vi "Fuel Injector Analysis Selection.vi"(8 "error in (no error)":errorcluster, 11 "Node Ptr":T1 format="%.0x") -> (0 "error out":errorcluster)   [LabVIEW 2019, in "Fuel Injector Analysis Addon System Explorer.lvlib"]
uses:
  Fuel Injector Analysis Addon System Explorer.lvlib
  <vilib>/NI VeriStand/Custom Device API/Custom Device Item Ref.ctl
  Addon Shared/Types/Analysis.Channels.Select.ctl
  <vilib>/NI VeriStand/Custom Device API/Custom Device API.lvlib
  Addon Shared/Fuel Injector Analysis Addon Shared.lvlib
panel:
  in  "Analysis":i32(listbox)=7
  in  "Reset":bool
  in  "Apply":bool
  in  "SHDocVw.IWebBrowser":refnum<k7>(container)
  in  "Header":cluster{"Section Name":string}={"Section Name"="Custom Device Item Settings"}
  in  "Description":string
  out "Name":string
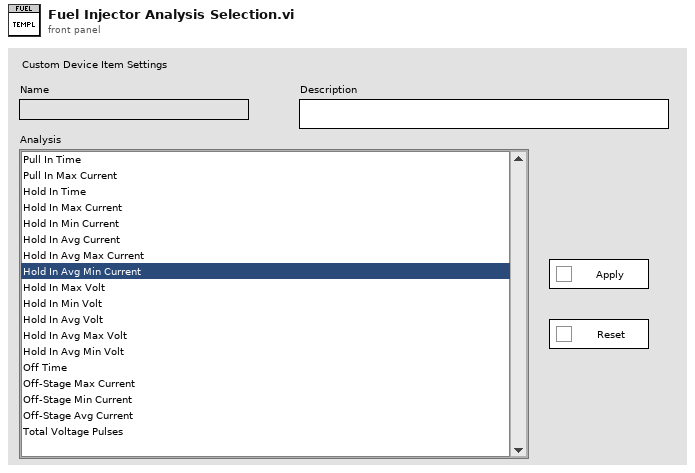
[diagram p1: front panel]
types:
  T1 = typedef "Custom Device API.lvlib/Custom Device Item Ref.ctl" = u64
  T2 = typedef "Custom Device API.lvlib/Custom Device Item Info.ctl" = cluster{"Name":string, "Is Channel":bool, "GUID":string, "Is Waveform":bool}
  T3 = typedef "Fuel Injector Analysis Addon Shared.lvlib/Analysis.Channels.Select.ctl" = cluster{"Pull In Time":bool, "Pull In Max Current":bool, "Pull In Max Voltage":bool, "Pull In Min Voltage":bool, "Pull In Avg Voltage":bool, "Hold Time":bool, "Hold Max Current":bool, "Hold Min Current":bool, "Hold Avg Current":bool, "Hold Max Voltage":bool, "Hold Min Voltage":bool, "Hold Avg Max Voltage":bool, "Hold Avg Min Voltage":bool, "Off Time":bool, "Off Max Current":bool, "Off Min Current":bool, "Off Avg Current":bool, "Off Max Voltage":bool, "Off Min Voltage":bool, "Off Avg Voltage":bool, "Total Voltage Pulses":bool, "Total Stage Time":bool}
  T4 = typedef "Custom Device API.lvlib/Custom Device Commands.ctl" = enum16{"Default", "Item renamed", "Shutdown", "Dynamic button pressed"}
  T5 = typedef "LVPoint32TypeDef.ctl" = cluster{"Horizontal":i32, "Vertical":i32}
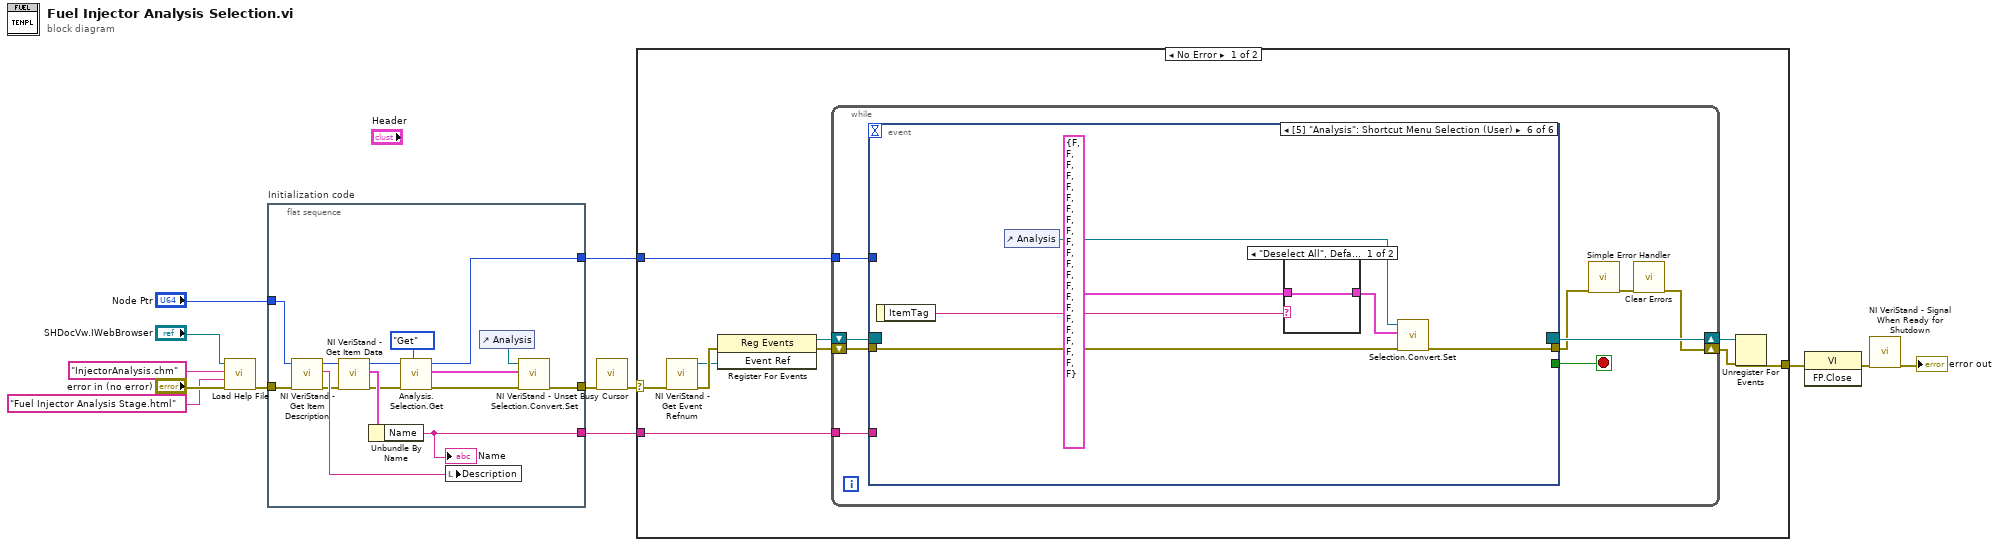
[diagram p0: block diagram]
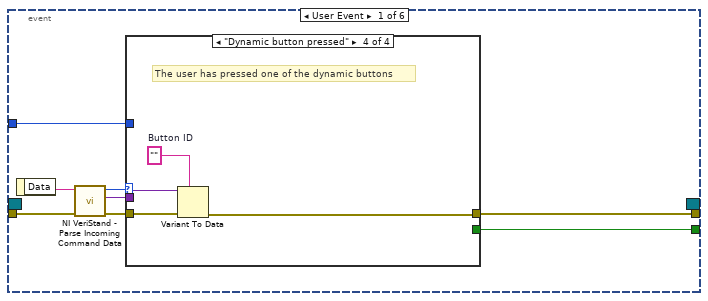
[diagram p2: hidden frame]
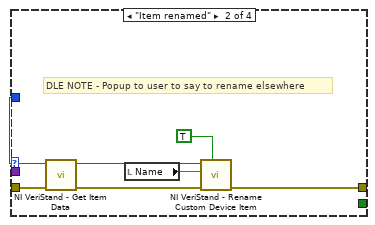
[diagram p4: hidden frame]
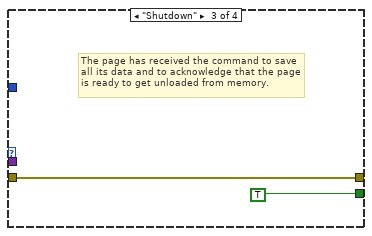
[diagram p5: hidden frame]
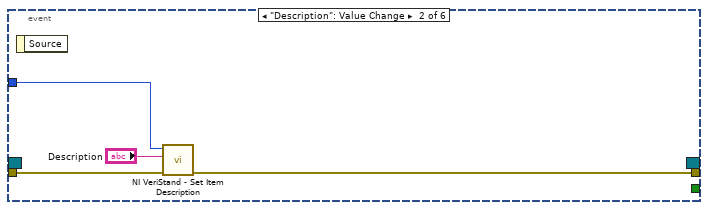
[diagram p6: hidden frame]
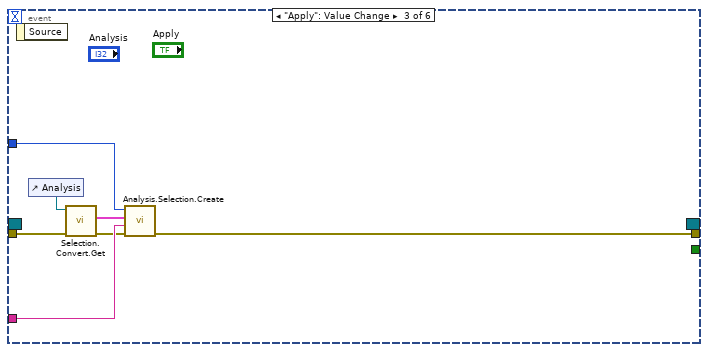
[diagram p7: hidden frame]
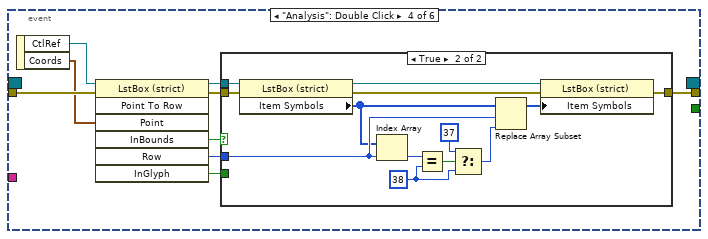
[diagram p8: hidden frame]
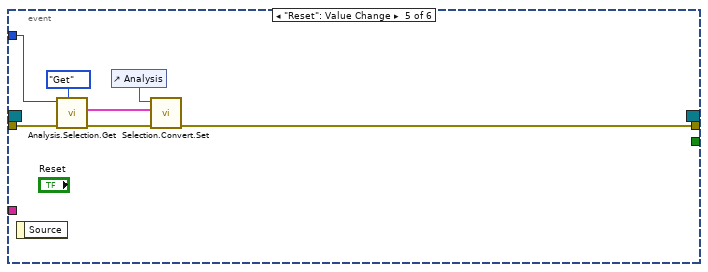
[diagram p10: hidden frame]
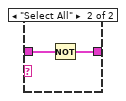
[diagram p11: hidden frame]
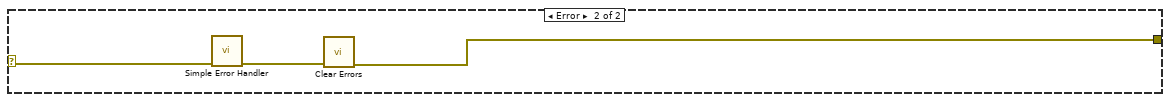
[diagram p12: hidden frame]
diagram:
  n1 = call "Load Help File.vi"("error in (no error)"="error in (no error)", "HTML File"="Fuel Injector Analysis Stage.html", "Main CHM File"="InjectorAnalysis.chm", "SHDocVw.IWebBrowser2"="SHDocVw.IWebBrowser") -> ("error out"=w6:errorcluster)  [unwired: 7 in]
  n2 = flat-sequence "Initialization code" {
    tunnel: w6 -> [w27]
    tunnel: [w15] -> w9
    tunnel: "Node Ptr" -> [w23]
    tunnel: [w20] -> w3
    tunnel: [w14] -> w2
    frame #0 {
      n3 = call <vilib>:"NI VeriStand - Get Item Description.vi"("error in (no error)"=w27, "Item Ref in"=w23) -> ("error out"=w25:errorcluster, "Description"=w26:string, "Item Ref out"=w28:T1)  [unwired: 7 out]
      n4 = call <vilib>:"NI VeriStand - Get Item Data.vi"("error in (no error)"=w25, "Item Ref in"=w28) -> ("error out"=w22:errorcluster, "Item Info"=w24:T2, "Item Ref out"=w21:T1)  [unwired: 7 out]
      n5 = Unbundle By Name(w24) -> ("Name"=w20:string)
      "Name" <- w20
      n6 = call "Analysis.Selection.Get.vi"("Action"=enum8{"Get", "Set"}."Get", "error in (no error)"=w22, "Item Ref in"=w21) -> ("error out"=w17:errorcluster, "Selections"=w18:T3, "Item Ref out"=w15:T1)  [unwired: 6 in]
      n7 = local write "Description"(w26) -> ()
      n8 = control-ref of="Analysis"() -> (w16:refnum<vi>)
      n9 = call "Selection.Convert.Set.vi"("error in (no error)"=w17, "Selections"=w18, "ListBox in"=w16) -> ("error out"=w14:errorcluster)  [unwired: 8 in]
    }
  }
  n10 = call <vilib>:"NI VeriStand - Unset Busy Cursor.vi"("error in (no error)"=w2) -> ("error out"=w10:errorcluster)  [unwired: 10 out]
  n11 = case shown="No Error" w10 {
    selector: w10 -> [w30 w122]
    tunnel: [w35 w120] -> w13
    tunnel: w9 -> [w31 _]
    tunnel: w3 -> [w29 _]
    frame No Error {
      n12 = call <vilib>:"NI VeriStand - Get Event Refnum.vi"("error in (no error)"=w30) -> ("error out"=w38:errorcluster, "Event Ref"=w34:refnum<user-event>)  [unwired: 9 out]
      n13 = register-events(error in=w38, w34) -> (reference out=w32:refnum<event-registration>, error out=w33:errorcluster)  [unwired: 1 in]
      n14 = while {
        tunnel: w31 -> [w43]
        shift-right: [w40] -> w36
        shift-left: w33 -> [w46]
        shift-right: [w47] -> w37
        shift-left: w32 -> [w45]
        tunnel: w29 -> [w39]
        stop <- w44 stop-if-true
        n15 = event shown="[5] \"Analysis\": Shortcut Menu Selection (User)" {
          selector: w45 -> [_ _ _ _ _ _]
          dyn-events: [_ _ _ _ _ _] -> w47
          timeout: _ -> [_ _ _ _ _ _]
          tunnel: w46 -> [w55 w72 w78 w83 w105 w114]
          tunnel: [w51 _ _ _ _ _] -> w44
          tunnel: [w50 w71 w74 w81 w107 w113] -> w42
          tunnel: w43 -> [w49 w73 w79 _ w104 _]
          tunnel: w39 -> [_ _ w80 _ _ _]
          event User Event {
            n16 = event-data() -> ("Data"=w54:string)  [unwired: 1 out]
            n17 = call <vilib>:"NI VeriStand - Parse Incoming Command Data.vi"("error in (no error)"=w55, "Incoming data"=w54) -> ("error out"=w53:errorcluster, "Outgoing data"=w48:variant, "Action"=w52:T4)  [unwired: 7 out]
            n18 = case shown="\"Dynamic button pressed\"" w52 {
              tunnel: w53 -> [w56 w63 w64 w69]
              tunnel: [_ _ TRUE _] -> w51
              tunnel: [w56 w60 w64 w66] -> w50
              tunnel: w49 -> [_ w62 _ _]
              tunnel: w48 -> [_ _ _ w68]
              frame "Default", Default {
              }
              frame "Item renamed" {
                # "DLE NOTE - Popup to user to say to rename elsewhere"
                n19 = call <vilib>:"NI VeriStand - Get Item Data.vi"("error in (no error)"=w63, "Item Ref in"=w62) -> ("error out"=w61:errorcluster, "Item Ref out"=w59:T1)  [unwired: 8 out]
                n20 = local read "Name"() -> (w58:string)
                n21 = call <vilib>:"NI VeriStand - Rename Custom Device Item.vi"("Force Rename (F)"=TRUE, "error in (no error)"=w61, "New Name"=w58, "Item Ref in"=w59) -> ("error out"=w60:errorcluster)  [unwired: 5 in, 2 out]
              }
              frame "Shutdown" {
                # "The page has received the command to save all its data and to acknowledge that the page is ready to get unloaded from memory."
              }
              frame "Dynamic button pressed" {
                w67 = ""  # Button ID
                # "The user has pressed one of the dynamic buttons"
                n22 = Variant To Data(error in=w69, type=w67, Variant=w68) -> (error out=w66:errorcluster)  [unwired: 1 out]
              }
            }
          }
          event "Description": Value Change {
            n23 = event-data() -> ()  [unwired: 2 out]
            n24 = call <vilib>:"NI VeriStand - Set Item Description.vi"("error in (no error)"=w72, "Description"="Description", "Item Ref in"=w73) -> ("error out"=w71:errorcluster)  [unwired: 8 out]
          }
          event "Apply": Value Change {
            n25 = event-data() -> ()  [unwired: 2 out]
            n26 = control-ref of="Analysis"() -> (w75:refnum<vi>)
            n27 = call "Selection.Convert.Get.vi"("error in (no error)"=w78, "ListBox in"=w75) -> ("error out"=w77:errorcluster, "Analysis Options"=w76:T3)  [unwired: 8 in]
            n28 = call "Analysis.Selection.Create.vi"("error in (no error)"=w77, "Name"=w80, "Analysis Options"=w76, "Item Ref in"=w79) -> ("error out"=w74:errorcluster)  [unwired: 7 in]
          }
          event "Analysis": Double Click {
            n29 = event-data() -> ("CtlRef"=w84:refnum<vi>, "Coords"=w82:T5)  [unwired: 1 out]
            n30 = invoke class="LstBox (strict)" method="Point To Row"(reference=w84, error in=w83, "Point"=w82) -> (reference out=w88:refnum<vi>, error out=w87:errorcluster, "InBounds"=w85:bool, "Row"=w86:i32, "InGlyph"=w89:bool)  [unwired: 4 in, 2 out]
            n31 = case shown="True" w85 {
              tunnel: w89 -> [_ _]
              tunnel: w88 -> [_ w103]
              tunnel: w87 -> [w90 w102]
              tunnel: w86 -> [_ w101]
              tunnel: [w90 w91] -> w81
              frame False {
              }
              frame True {
                w98 = 38
                n32 = property class="LstBox (strict)"(reference=w103, error in=w102) -> (reference out=w94:refnum<vi>, error out=w93:errorcluster, "Item Symbols"=w96:i32[])
                n33 = Index Array(array=w96, index=w101) -> (element=w100:i32)
                n34 = Equal?(x=w100, y=w98) -> (x = y?=w99:bool)
                n35 = Select(t=37, s=w99, f=w98) -> (s? t:f=w95:i32)
                n36 = Replace Array Subset(array=w96, new element=w95, index=w101) -> (w92:i32[])
                n37 = property class="LstBox (strict)"(reference=w94, error in=w93, "Item Symbols"=w92) -> (error out=w91:errorcluster)  [unwired: 1 out]
              }
            }
          }
          event "Reset": Value Change {
            n38 = event-data() -> ()  [unwired: 2 out]
            n39 = call "Analysis.Selection.Get.vi"("Action"=enum8{"Get", "Set"}."Get", "error in (no error)"=w105, "Item Ref in"=w104) -> ("error out"=w108:errorcluster, "Selections"=w106:T3)  [unwired: 6 in, 1 out]
            n40 = control-ref of="Analysis"() -> (w109:refnum<vi>)
            n41 = call "Selection.Convert.Set.vi"("error in (no error)"=w108, "Selections"=w106, "ListBox in"=w109) -> ("error out"=w107:errorcluster)  [unwired: 8 in]
          }
          event "Analysis": Shortcut Menu Selection (User) {
            n42 = event-data() -> ("ItemTag"=w111:string)  [unwired: 1 out]
            n43 = control-ref of="Analysis"() -> (w112:refnum<vi>)
            n44 = case shown="\"Deselect All\", Default" w111 {
              tunnel: [w117 w119] -> w116
              tunnel: T3 {"Pull In Time"=FALSE, "Pull In Max Current"=FALSE, "Pull In Max Voltage"=FALSE, "Pull In Min Voltage"=FALSE, "Pull In Avg Voltage"=FALSE, "Hold Time"=FALSE, "Hold Max Current"=FALSE, "Hold Min Current"=FALSE, "Hold Avg Current"=FALSE, "Hold Max Voltage"=FALSE, "Hold Min Voltage"=FALSE, "Hold Avg Max Voltage"=FALSE, "Hold Avg Min Voltage"=FALSE, "Off Time"=FALSE, "Off Max Current"=FALSE, "Off Min Current"=FALSE, "Off Avg Current"=FALSE, "Off Max Voltage"=FALSE, "Off Min Voltage"=FALSE, "Off Avg Voltage"=FALSE, "Total Voltage Pulses"=FALSE, "Total Stage Time"=FALSE} ("Selections") -> [w117 w118]
              frame "Deselect All", Default {
              }
              frame "Select All" {
                n45 = Not(x=w118) -> (.not. x?=w119:T3)
              }
            }
            n46 = call "Selection.Convert.Set.vi"("error in (no error)"=w114, "Selections"=w116, "ListBox in"=w112) -> ("error out"=w113:errorcluster)  [unwired: 8 in]
          }
        }
        n47 = call <vilib>:"Simple Error Handler.vi"("error in (no error)"=w42) -> ("error out"=w41:errorcluster)  [unwired: 1 in, 7 out]
        n48 = call <vilib>:"Clear Errors.vi"("error in (no error)"=w41) -> ("error out"=w40:errorcluster)  [unwired: 1 in, 5 out]
      }
      n49 = Unregister For Events(event registration refnum=w37, error in=w36) -> (error out=w35:errorcluster)
    }
    frame Error {
      n50 = call <vilib>:"Simple Error Handler.vi"("error in (no error)"=w122) -> ("error out"=w121:errorcluster)  [unwired: 1 in, 7 out]
      n51 = call <vilib>:"Clear Errors.vi"("error in (no error)"=w121) -> ("error out"=w120:errorcluster)  [unwired: 1 in, 5 out]
    }
  }
  n52 = invoke class="VI" method="FP.Close"(error in=w13) -> (error out=w12:errorcluster)  [unwired: 2 in, 2 out]
  n53 = call <vilib>:"NI VeriStand - Signal When Ready for Shutdown.vi"("error in (no error)"=w12) -> ("error out"=→"error out":errorcluster)  [unwired: 10 out]
